vi "Save Baseline Image.vi"(8 "error in (no error)":errorcluster, 10 "Baseline Image Path":path, 11 "Baseline Image":T1) -> (0 "error out":errorcluster, 3 "Baseline Image Out":T1)   [LabVIEW 2011]
uses:
  <vilib>/vision/Image Controls.llb/IMAQ Image.ctl
  DepthSense/IT WORKS SO SUCK IT/DepthSense Global Status.vi
  <vilib>/vision/NI_Vision_Development_Module.lvlib
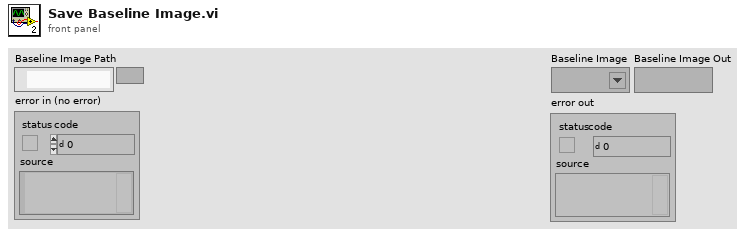
[diagram p1: front panel]
types:
  T1 = typedef "IMAQ Image.ctl" = refnum<image>
  T2 = typedef "Image Type" = u32
  T3 = cluster{"Camera Version":string, "Image Height":i32, "Image Width":i32, "Minimum Framerate":i32, "Maximum Framerate":i32, "Framerate":i32, "Close Mode":bool, "Denoising":bool, "Leakage Algorithm":bool, "Anti-Aliasing":bool, "Camera Status":i32, "API Version":string, "Light Intensity":i32, "Confidence Threshold":u16, "Range":sgl}
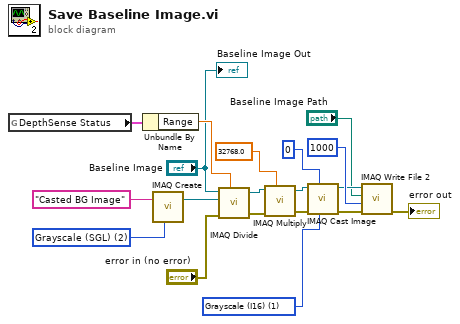
[diagram p0: block diagram]
diagram:
  w5 = T2 2 items=["Grayscale (U8)", "Grayscale (I16)", "Grayscale (SGL)", "Complex (CSG)", "RGB (U32)", "HSL (U32)", "RGB (U64)", "Grayscale (U16)"] ("Image Type")
  w12 = T2 1 items=["Grayscale (U8)", "Grayscale (I16)", "Grayscale (SGL)", "Complex (CSG)", "RGB (U32)", "HSL (U32)", "RGB (U64)", "Grayscale (U16)"] ("Image Type")
  n1 = global read "DepthSense Global Status.vi" "DepthSense Status"() -> (w19:T3)
  n2 = Unbundle By Name(w19) -> ("Range"=w18:sgl)
  n3 = call "IMAQ Create"("Image Name"="Casted BG Image", "Image Type"=w5) -> ("New Image"=w3:T1)  [unwired: 3 in, 1 out]
  n4 = call "IMAQ Divide"("Image Src A"="Baseline Image", "Constant"=w18, "Image Dst"=w3, "error in (no error)"="error in (no error)") -> ("Image Dst Out"=w16:T1, "error out"=w17:errorcluster)  [unwired: 3 in]
  n5 = call "IMAQ Multiply"("Image Src A"=w16, "Constant"=sgl 32768.0, "error in (no error)"=w17) -> ("Image Dst Out"=w1:T1, "error out"=w13:errorcluster)  [unwired: 4 in]
  n6 = call "IMAQ Cast Image"("Image Type"=w12, "# Shifts"=0, "error in (no error)"=w13, "Image Src"=w1) -> ("error out"=w8:errorcluster, "Image Dst Out"=w9:T1)  [unwired: 6 in]
  n7 = call-poly "IMAQ Write File 2"("error in (no error)"=w8, "Image Quality"=u32 1000, "File Path"="Baseline Image Path", "Image"=w9) -> ("error out"=→"error out":errorcluster)  [unwired: 6 in, 1 out]
  "Baseline Image Out" <- "Baseline Image"
